vi "sweep_string_2_vector.vi"(1 "Field string":string="-40:1:40" caption="sweep string in") -> (0 "vector out":dbl[](array[numeric]))   [LabVIEW 2015]
uses:
  polys/poly_linspace_DBL.vi
  <vilib>/GPower/Numeric/Library/Round/RoundDBL.vi
  <userlib>/_OpenG.lib/array/array.llb/Remove Duplicates from 1D Array (DBL)__ogtk.vi
  <vilib>/GPower/Numeric/GPNumeric.lvlib
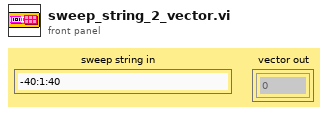
[diagram p1: front panel]
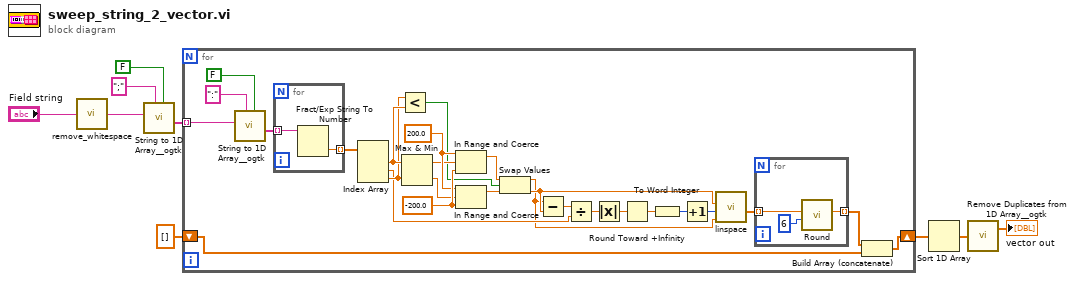
[diagram p0: block diagram]
diagram:
  n1 = call "remove_whitespace.vi"("string in"="Field string") -> ("string out"=w3:string)  [unwired: 4 in]
  n2 = call <userlib>:"String to 1D Array__ogtk.vi"("ignore duplicate delimiters? (F=No)"=FALSE, "delimiter (Tab)"=";" ("Search string"), "string"=w3) -> ("Array of Strings"=w7:string[])  [unwired: 8 in]
  n3 = for {
    tunnel: w7 -> [w18] mode=indexing
    shift-right: [w20] -> w2
    shift-left: dbl[] [] -> [w19]
    w33 = -200.0 ("upper limit")
    w32 = 200.0 ("upper limit")
    n4 = call <userlib>:"String to 1D Array__ogtk.vi"("ignore duplicate delimiters? (F=No)"=FALSE, "delimiter (Tab)"=":" ("Search string"), "string"=w18) -> ("Array of Strings"=w16:string[])  [unwired: 8 in]
    n5 = for {
      tunnel: w16 -> [w41] mode=indexing
      tunnel: [w40] -> w36 mode=indexing
      n6 = Fract/Exp String To Number(string=w41) -> (number=w40:dbl)  [unwired: 3 in, 1 out]
    }
    n7 = Index Array(array=w36) -> (element #1=w29:dbl, element #2=w23:dbl, element #3=w28:dbl)  [unwired: 3 in]
    n8 = Less?(x=w28, y=w29) -> (x < y?=w26:bool)
    n9 = Max & Min(x=w29, y=w28) -> (max(x,y)=w31:dbl, min(x,y)=w30:dbl)
    n10 = In Range and Coerce(upper limit=w32, x=w31, lower limit=w33) -> (coerced(x)=w34:dbl)  [unwired: 1 out]
    n11 = In Range and Coerce(upper limit=w32, x=w30, lower limit=w33) -> (coerced(x)=w35:dbl)  [unwired: 1 out]
    n12 = Swap Values(12:w34, 13:w26, 14:w35) -> (1:w12:dbl, 3:w13:dbl)
    n13 = Subtract(x=w12, y=w13) -> (x-y=w24:dbl)
    n14 = Divide(x=w24, y=w23) -> (x/y=w22:dbl)
    n15 = Absolute Value(x=w22) -> (abs(x)=w21:dbl)
    n16 = Round Toward +Infinity(x=w21) -> (ceil(x): smallest int >= x=w27:dbl)
    n17 = To Word Integer(number=w27) -> (16bit integer=w25:i16)
    n18 = Increment(x=w25) -> (x+1=w11:i16)
    n19 = call-poly "linspace.vi"("xN"=w12, "N"=w11, "x0"=w13) -> ("linspace out"=w10:dbl[])  [unwired: 8 in]
    n20 = for {
      tunnel: w10 -> [w39] mode=indexing
      tunnel: [w38] -> w14 mode=indexing
      n21 = call-poly <vilib>:"Round.vi"("Decimal places"=i8 6, "Number"=w39) -> ("Rounded number"=w38:dbl)  [unwired: 5 in]
    }
    n22 = Build Array (concatenate)(w14, w19) -> (w20:dbl[])
  }
  n23 = Sort 1D Array(array=w2) -> (sorted array=w1:dbl[])
  n24 = call-poly <userlib>:"Remove Duplicates from 1D Array__ogtk.vi"("Input Array"=w1) -> ("Output Array"=→"vector out":dbl[])  [unwired: 1 out]
